vi "niWLAN - 80211agn Spectral Flatness Index.vi"(0 "spectral flatness upper mask":T1, 5 "spectral flatness Trace":T1, 7 "spectral flatness Lower mask":T1, 11 "error in (no error)":errorcluster) -> (4 "Least Spectral Flatness Margin":dbl, 6 "Spectral Flatness Margin Subcarrier Index":i32, 15 "error out":errorcluster)   [LabVIEW 2012]
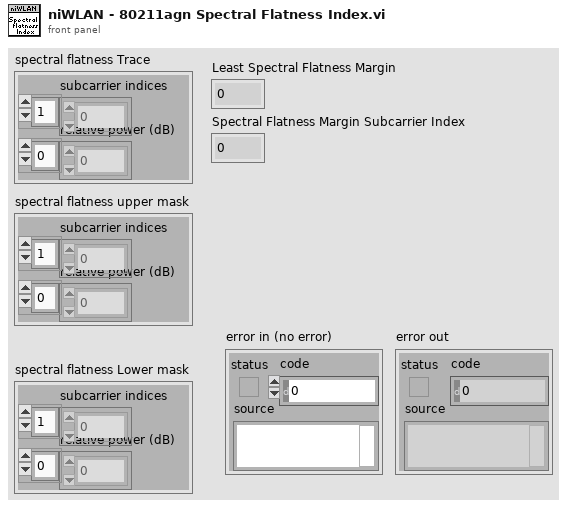
[diagram p1: front panel]
types:
  T1 = cluster{"subcarrier indices":i32[], "relative power (dB)":dbl[]}
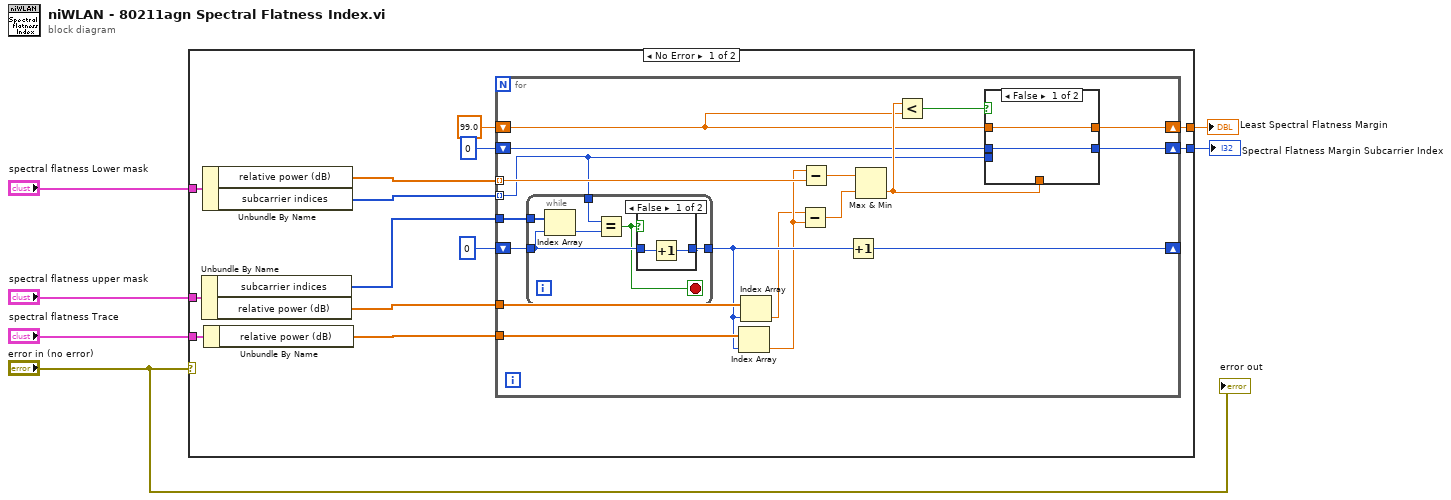
[diagram p0: block diagram]
diagram:
  n1 = case shown="No Error" "error in (no error)" {
    tunnel: "spectral flatness Lower mask" -> [w19 _]
    tunnel: "spectral flatness Trace" -> [w18 _]
    tunnel: "spectral flatness upper mask" -> [w17 _]
    tunnel: [w8 _] -> w3
    tunnel: [w7 _] -> w2
    frame No Error {
      n2 = Unbundle By Name(w17) -> ("subcarrier indices"=w15:i32[], "relative power (dB)"=w10:dbl[])
      n3 = Unbundle By Name(w19) -> ("relative power (dB)"=w13:dbl[], "subcarrier indices"=w16:i32[])
      n4 = Unbundle By Name(w18) -> ("relative power (dB)"=w9:dbl[])
      n5 = for {
        tunnel: w16 -> [w22] mode=indexing
        tunnel: w15 -> [w37]
        shift-right: [w36] -> _
        shift-left: 0 ("index") -> [w35]
        tunnel: w13 -> [w34] mode=indexing
        shift-right: [w27] -> w8
        shift-left: 99.0 ("element") -> [w23]
        shift-right: [w25] -> w7
        shift-left: 0 ("index") -> [w24]
        tunnel: w10 -> [w31]
        tunnel: w9 -> [w30]
        n6 = while {
          tunnel: w37 -> [w43]
          tunnel: w35 -> [w41]
          tunnel: [w40] -> w26
          tunnel: w22 -> [w39]
          stop <- w38 stop-if-true
          n7 = Index Array(array=w43, index=w41) -> (element=w42:i32)
          n8 = Equal?(x=w39, y=w42) -> (x = y?=w38:bool)
          n9 = case shown="False" w38 {
            tunnel: w41 -> [w45 w46]
            tunnel: [w44 w46] -> w40
            frame False {
              n10 = Increment(x=w45) -> (x+1=w44:i32)
            }
            frame True {
            }
          }
        }
        n11 = Index Array(array=w30, index=w26) -> (element=w21:dbl)
        n12 = Index Array(array=w31, index=w26) -> (element=w20:dbl)
        n13 = Subtract(x=w20, y=w21) -> (x-y=w32:dbl)
        n14 = Subtract(x=w21, y=w34) -> (x-y=w33:dbl)
        n15 = Increment(x=w26) -> (x+1=w36:i32)
        n16 = Max & Min(x=w33, y=w32) -> (min(x,y)=w28:dbl)  [unwired: 1 out]
        n17 = Less?(x=w28, y=w23) -> (x < y?=w29:bool)
        n18 = case shown="False" w29 {
          tunnel: w28 -> [_ w50]
          tunnel: [w47 w50] -> w27
          tunnel: w22 -> [_ w49]
          tunnel: [w48 w49] -> w25
          tunnel: w24 -> [w48 _]
          tunnel: w23 -> [w47 _]
          frame False {
          }
          frame True {
          }
        }
      }
    }
    frame Error {
    }
  }
  "Least Spectral Flatness Margin" <- w3
  "Spectral Flatness Margin Subcarrier Index" <- w2
  "error out" <- "error in (no error)"
